vi "Enqueue.vi"(6 "Priority?":bool, 8 "error in (no error)":errorcluster, 9 "Data":variant, 10 "Message":string) -> (0 "error out":errorcluster)   [LabVIEW 2017, in "Messaging Library.lvlib"]
uses:
  Messaging Library.lvlib
  Controls/Msg TypeDef.ctl
  Controls/Q FGV States.ctl
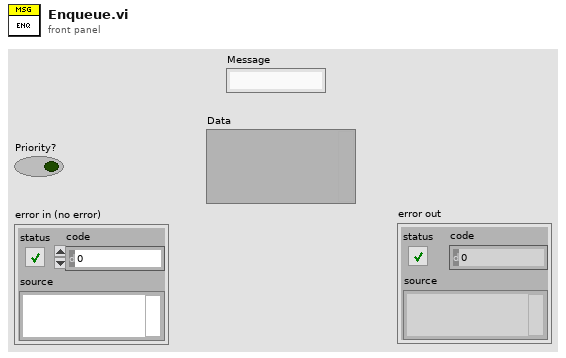
[diagram p1: front panel]
types:
  T1 = typedef "Messaging Library.lvlib/Q FGV States.ctl" = enum16{"Set", "Get"}
  T2 = typedef "Messaging Library.lvlib/Msg TypeDef.ctl" = cluster{"Message":string, "Data":variant}
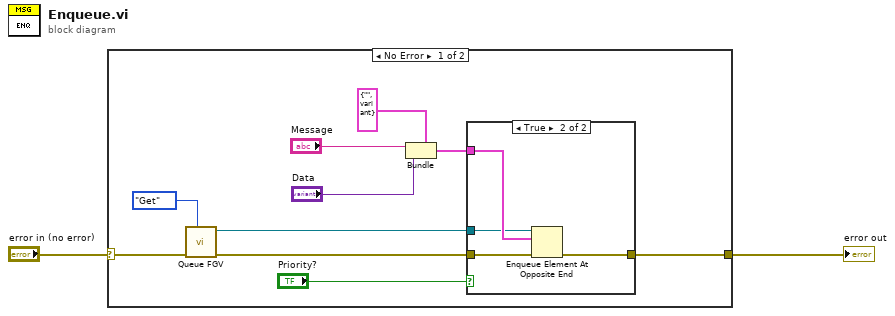
[diagram p0: block diagram]
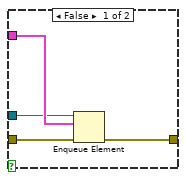
[diagram p2: hidden frame]
diagram:
  n1 = case shown="No Error" "error in (no error)" {
    selector: "error in (no error)" -> [w6 w21]
    tunnel: [w11 w21] -> w1
    frame No Error {
      n2 = call "Queue FGV.vi"("States"=Q_FGV_States."Get", "error in (no error)"=w6) -> ("error out"=w5:errorcluster, "Message Q Out"=w3:refnum<queue>)  [unwired: 8 in]
      n3 = Bundle(cluster=T2 {"Message"="", "Data"=variant} ("Message Cluster"), "Message"="Message", "Data"="Data") -> (w10:T2)
      n4 = case shown="True" "Priority?" {
        tunnel: w5 -> [w16 w20]
        tunnel: [w15 w19] -> w11
        tunnel: w10 -> [w14 w18]
        tunnel: w3 -> [w13 w17]
        frame False {
          n5 = Enqueue Element(queue=w13, element=w14, error in (no error)=w16) -> (error out=w15:errorcluster)  [unwired: 1 in, 2 out]
        }
        frame True {
          n6 = Enqueue Element At Opposite End(queue=w17, element=w18, error in (no error)=w20) -> (error out=w19:errorcluster)  [unwired: 1 in, 2 out]
        }
      }
    }
    frame Error {
    }
  }
  "error out" <- w1
